vi "Status Control Parameters.vi"(0 "VISA resource name":refnum<visa-resource-name>, 5 "Loop (0: 1)":u16(ring) items=["1", "2"], 11 "error in (no error)":errorcluster) -> (3 "Loop 1 Tuning Status":bool, 4 "VISA resource name out":refnum<visa-resource-name>, 6 "Gain (P)":dbl min=0.0 max=1000.0 step=0.1 format="%.1f", 8 "Reset (I)":dbl min=0.0 max=1000.0 step=0.1 format="%.1f", 10 "Rate (D)":dbl min=0.0 max=1000.0 step=0.1 format="%.1f", 13 "Loop 1 Heater Range":u16(ring) items=["Off", "Low (0.5W)", "Med (5W)", "High (50W)"], 14 "Manual Output (0.000 %)":dbl min=0.0 max=100.0 step=0.001 format="%.3f", 15 "error out":errorcluster)   [LabVIEW 2013, in "Lake Shore Cryotronics 331.lvlib"]
doc: "This VI indicates the status of the control parameters for the selected loop."
uses:
  Lake Shore Cryotronics 331.lvlib
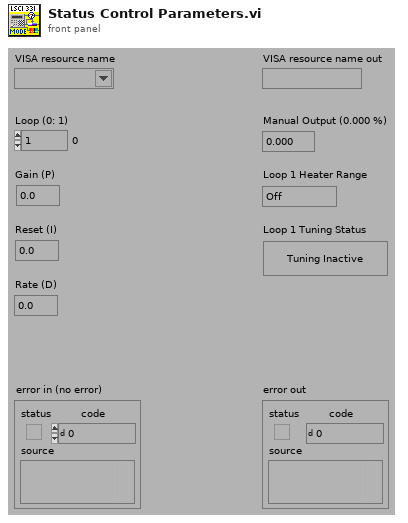
[diagram p1: front panel]
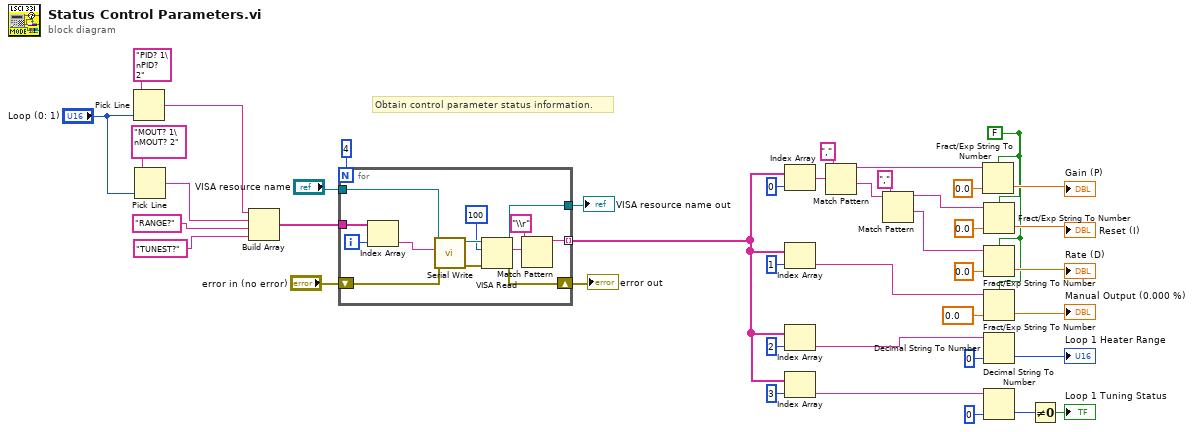
[diagram p0: block diagram]
diagram:
  w1 = FALSE ("use system decimal point (T)")
  # "Obtain control parameter status information."
  n1 = Pick Line(multi-line string="PID? 1\nPID? 2", line index="Loop (0: 1)") -> (output string=w33:string)  [unwired: 1 in]
  n2 = Pick Line(multi-line string="MOUT? 1\nMOUT? 2", line index="Loop (0: 1)") -> (output string=w32:string)  [unwired: 1 in]
  n3 = Build Array(w33, w32, "RANGE?", "TUNEST?") -> (w31:string[])
  n4 = for {
    N: 4 -> [_]
    tunnel: w31 -> [w44]
    shift-right: [w49] -> w37
    shift-left: "error in (no error)" -> [w50]
    tunnel: [w48] -> w38
    tunnel: "VISA resource name" -> [w47]
    tunnel: [w45] -> w7 mode=indexing
    i -> [w51]
    n5 = Index Array(array=w44, index=w51) -> (element=w43:string)
    n6 = call "Serial Write.vi"("error in (no error)"=w50, "Write Buffer (\"\")"=w43, "VISA resource name"=w47) -> ("error out"=w54:errorcluster, "VISA resource name out"=w55:refnum<visa-resource-name>)  [unwired: 6 in, 1 out]
    n7 = VISA Read(VISA resource name=w55, byte count=100, error in (no error)=w54) -> (VISA resource name out=w48:refnum<visa-resource-name>, read buffer=w52:string, error out=w49:errorcluster)  [unwired: 1 out]
    n8 = Match Pattern(string=w52, regular expression="\\r") -> (before substring=w45:string)  [unwired: 1 in, 3 out]
  }
  "error out" <- w37
  "VISA resource name out" <- w38
  n9 = Index Array(array=w7, index=0) -> (element=w26:string)
  n10 = Index Array(array=w7, index=1) -> (element=w12:string)
  n11 = Index Array(array=w7, index=2) -> (element=w10:string)
  n12 = Index Array(array=w7, index=3) -> (element=w4:string)
  n13 = Match Pattern(string=w26, regular expression=",") -> (before substring=w20:string, after substring=w24:string)  [unwired: 1 in, 2 out]
  n14 = Match Pattern(string=w24, regular expression=",") -> (before substring=w19:string, after substring=w18:string)  [unwired: 1 in, 2 out]
  n15 = Fract/Exp String To Number(use system decimal point (T)=w1, string=w20, default (0 dbl)=0.0 ("default (0L)")) -> (number=→"Gain (P)":dbl)  [unwired: 1 in, 1 out]
  n16 = Fract/Exp String To Number(use system decimal point (T)=w1, string=w19, default (0 dbl)=0.0 ("default (0L)")) -> (number=→"Reset (I)":dbl)  [unwired: 1 in, 1 out]
  n17 = Fract/Exp String To Number(use system decimal point (T)=w1, string=w18, default (0 dbl)=0.0 ("default (0L)")) -> (number=→"Rate (D)":dbl)  [unwired: 1 in, 1 out]
  n18 = Fract/Exp String To Number(use system decimal point (T)=w1, string=w12, default (0 dbl)=0.0 ("default (0L)")) -> (number=→"Manual Output (0.000 %)":dbl)  [unwired: 1 in, 1 out]
  n19 = Decimal String To Number(string=w10, default (0L)=u16 0) -> (number=→"Loop 1 Heater Range":u16)  [unwired: 1 in, 1 out]
  n20 = Decimal String To Number(string=w4, default (0L)=u16 0) -> (number=w3:u16)  [unwired: 1 in, 1 out]
  n21 = Not Equal To 0?(x=w3) -> (x != 0?=→"Loop 1 Tuning Status":bool)
